vi "Center Frame.vi"(8 "error in (no error)":errorcluster, 11 "VI in":refnum<vi>) -> (0 "error out":errorcluster)   [LabVIEW 2017]
uses:
  <vilib>/Utility/miscctls.llb/LVPointTypeDef.ctl
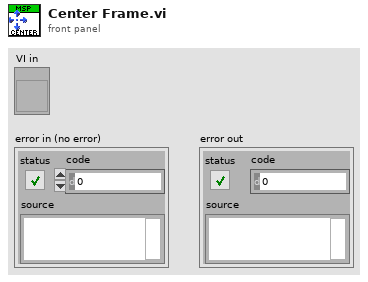
[diagram p1: front panel]
types:
  T1 = typedef "LVPointTypeDef.ctl" = cluster{"Horizontal":i16, "Vertical":i16}
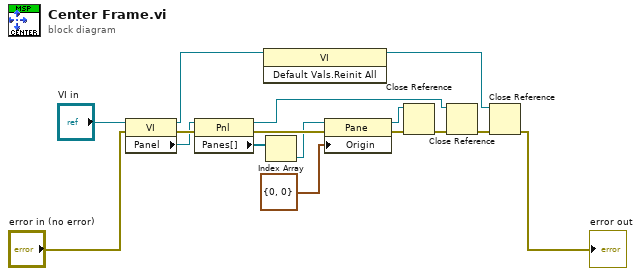
[diagram p0: block diagram]
diagram:
  n1 = property class="VI"(reference="VI in", error in="error in (no error)") -> (reference out=w7:refnum<vi>, error out=w8:errorcluster, "Panel"=w2:refnum<vi>)
  n2 = property class="Pnl"(reference=w2, error in=w8) -> (reference out=w6:refnum<vi>, error out=w9:errorcluster, "Panes[]"=w3:refnum<vi>[])
  n3 = invoke class="VI" method="Default Vals.Reinit All"(reference=w7) -> (reference out=w14:refnum<vi>)  [unwired: 2 in, 2 out]
  n4 = Index Array(array=w3) -> (element=w4:refnum<vi>)  [unwired: 1 in]
  n5 = property class="Pane"(reference=w4, error in=w9, "Origin"=T1 {"Horizontal"=0, "Vertical"=0}) -> (reference out=w5:refnum<vi>, error out=w10:errorcluster)
  n6 = Close Reference(reference=w5, error in (no error)=w10) -> (error out=w11:errorcluster)
  n7 = Close Reference(reference=w6, error in (no error)=w11) -> (error out=w12:errorcluster)
  n8 = Close Reference(reference=w14, error in (no error)=w12) -> (error out=→"error out":errorcluster)
